vi "(Un)tag Keys.vi"(5 "Key name/Regex":string, 6 "Tag (T)\\Untag (F) [T]":bool=TRUE, 7 "Section name/Regex":string, 8 "error in (no error)":errorcluster, 9 "Use Key Regex? [F]":bool, 10 "Use Section Regex? [F]":bool, 11 "Carya Config in":refnum<class "Carya Config.lvclass">) -> (0 "error out":errorcluster, 3 "Carya Config out":refnum<class "Carya Config.lvclass">)   [LabVIEW 2013, in "Carya Config.lvclass"]
doc: "Copyright 2018, Carya Automatisering, Wiebe Walstra."
uses:
  Carya Config.lvclass
  CConfig Object/Data.ctl
  CConfig Object/CConfig Object.lvclass
  CConfig Object/Add Results Query/Add Results Query.lvclass
  CConfig Object/Set Query/Set Query.lvclass
panel:
  out "Key names":string[](array[string])
  out "Section names":string[](array[string])
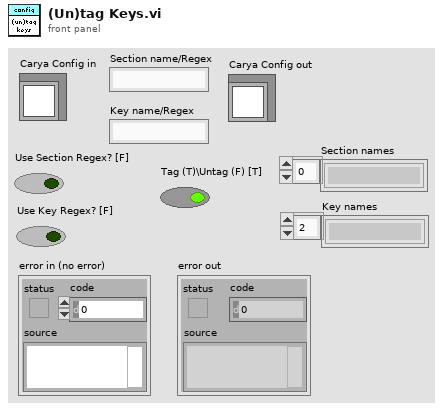
[diagram p1: front panel]
types:
  T1 = typedef "CConfig Object.lvclass/Data.ctl" = enum16{"pre", "name", "middle", "value", "post", "newline", "persistant", "tagged", "type"}
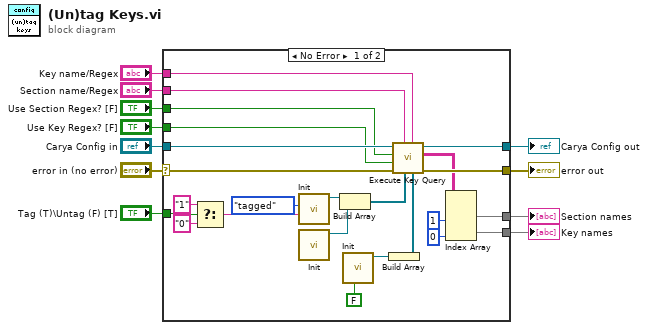
[diagram p0: block diagram]
diagram:
  n1 = case shown="No Error" "error in (no error)" {
    selector: "error in (no error)" -> [w35 w37]
    tunnel: [w33 w37] -> w10
    tunnel: [w32 w36] -> w8
    tunnel: "Carya Config in" -> [w31 w36]
    tunnel: "Section name/Regex" -> [w18 _]
    tunnel: "Use Section Regex? [F]" -> [w16 _]
    tunnel: "Key name/Regex" -> [w17 _]
    tunnel: "Use Key Regex? [F]" -> [w15 _]
    tunnel: "Tag (T)\\Untag (F) [T]" -> [w34 _]
    tunnel: [w30 _] -> w2
    tunnel: [w29 _] -> w1
    frame No Error {
      n2 = Select(t="1" ("Value"), s=w34, f="0") -> (s? t:f=w19:string)
      n3 = call "Init.vi"("Value"=w19, "Data [value]"=Data."tagged" ("Data")) -> ("Set Query out"=w27:refnum<class "Set Query.lvclass">)  [unwired: 8 in, 1 out]
      n4 = call "Init.vi"() -> ("Find First Query out"=w26:refnum<class "Add Results Query.lvclass">)  [unwired: 10 in, 1 out]
      n5 = Build Array(w27, w26) -> (w12:refnum<class "CConfig Query.lvclass">[])
      n6 = call "Init.vi"("Concatenate\\Build [T, Concatenate]"=FALSE ("Concatenate\\Build [T, Concatenate]")) -> ("Find First Query out"=w14:refnum<class "Add Results Query.lvclass">)  [unwired: 9 in, 1 out]
      n7 = Build Array(w14) -> (w13:refnum<class "Add Results Query.lvclass">[])
      n8 = call-dynamic "Execute Key Query.vi"("Section queries"=w13, "Key name"=w17, "Key queries"=w12, "Section name"=w18, "error in (no error)"=w35, "Use Key Regex? [F]"=w15, "Use Section Regex? [F]"=w16, "Carya Config in"=w31) -> ("error out"=w33:errorcluster, "Results"=w24:string[][], "Carya Config out"=w32:refnum<class "Carya Config.lvclass">)  [unwired: 1 in]
      n9 = Index Array(array=w24, index (col) #1=1 ("disabled index (col)"), index (col) #2=0 ("index (col)")) -> (element #1=w30:string[], element #2=w29:string[])  [unwired: 2 in]
    }
    frame Error {
    }
  }
  "error out" <- w10
  "Carya Config out" <- w8
  "Section names" <- w2
  "Key names" <- w1
